vi "Create.vi"(8 "error in (no error)":errorcluster, 9 "Configuration File Path":path=path "") -> (0 "error out":errorcluster, 3 "Execution UI Out":refnum<class "Execution UI V2.lvclass">)   [LabVIEW 2020, in "Execution UI V2.lvclass"]
uses:
  Execution UI V2.lvclass
  Execution UI V2.lvclass/Execution UI V2.ctl
  Application Framework/Process Classes/Process/Process.lvclass
  C:/Git/astemes-lunit/source/Application Framework/Process Classes/Process/Process.lvclass
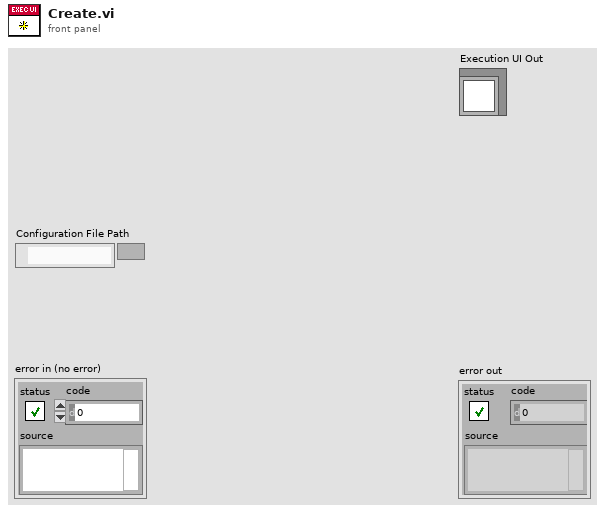
[diagram p1: front panel]
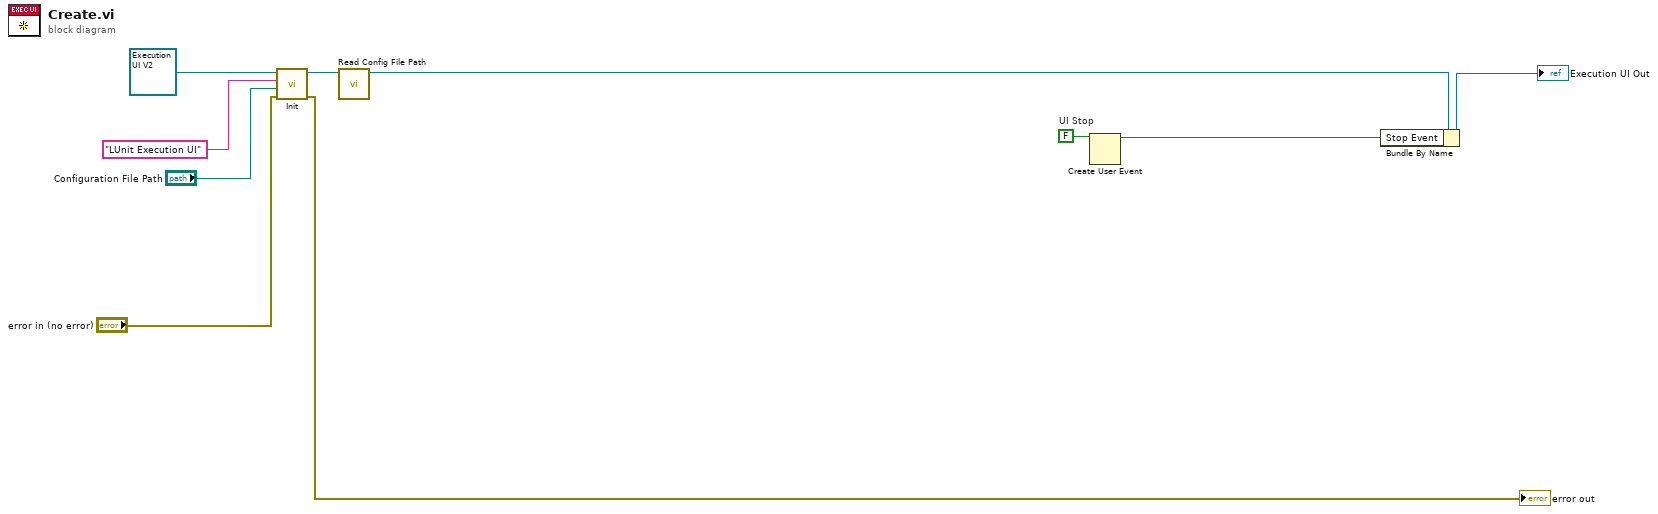
[diagram p0: block diagram]
diagram:
  w5 = FALSE  # UI Stop
  n1 = call-dynamic "Init.vi"("error in (no error)"="error in (no error)", "Config File Path"="Configuration File Path", "Name"="LUnit Execution UI", "Process In"=refnum<class "Execution UI V2.lvclass"> refnum ("Execution UI In")) -> ("error out"=→"error out":errorcluster, "Process Out"=w3:refnum<class "Execution UI V2.lvclass">)  [unwired: 6 in]
  n2 = call "Read Config File Path.vi"("Process In"=w3) -> ("Process Out"=w2:refnum<class "Execution UI V2.lvclass">)  [unwired: 9 in, 1 out]
  n3 = Create User Event(user event datatype=w5) -> (user event=w4:refnum<user-event>)  [unwired: 1 in, 1 out]
  n4 = Bundle By Name(cluster=w2, "Stop Event"=w4) -> (→"Execution UI Out":refnum<class "Execution UI V2.lvclass">)
